vi "Assign switches.vi"(8 "error in (no error)":errorcluster, 10 "Channel Array In":T1=[{"Channel x"="x6", "Channel y"="y1"}, {"Channel x"="x2", "Channel y"="y5"}]) -> (0 "error out":errorcluster, 2 "Channel Array Out":T1=[{"Channel x"="xA6", "Channel y"="yA1"}, {"Channel x"="comB6", "Channel y"="chB6"}, {"Channel x"="comD1", "Channel y"="chD1"}, {"Channel x"="xA2", "Channel y"="yA5"}, {"Channel x"="comC2", "Channel y"="chC2"}, {"Channel x"="comD5", "Channel y"="chD5"}])   [LabVIEW 2016, in "pickering.lvclass"]
uses:
  pickering.lvclass
  Typedefs/Channels-Array.ctl
  Typedefs/Channel-Cluster.ctl
  Typedefs/ChannelX-ComboBox.ctl
  Typedefs/ChannelY-ComboBox.ctl
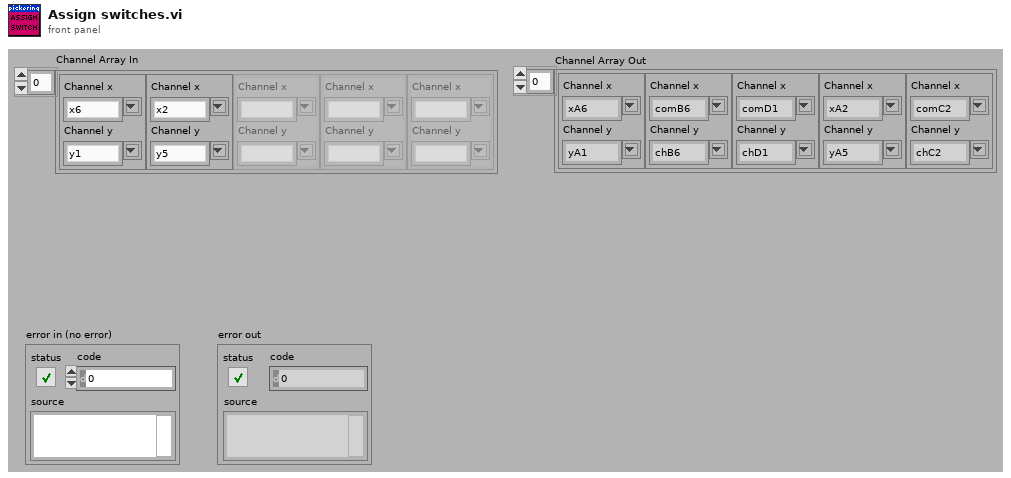
[diagram p1: front panel]
types:
  T1 = typedef "pickering.lvclass/Channels-Array.ctl" = T2[]
  T2 = typedef "pickering.lvclass/Channel-Cluster.ctl" = cluster{"Channel x":T3, "Channel y":T4}
  T3 = typedef "pickering.lvclass/ChannelX-ComboBox.ctl" = string
  T4 = typedef "pickering.lvclass/ChannelY-ComboBox.ctl" = string
  T5 = cluster{"result string":string, "result string":string}
  T6 = cluster{"result string":string, "result string":string}[]
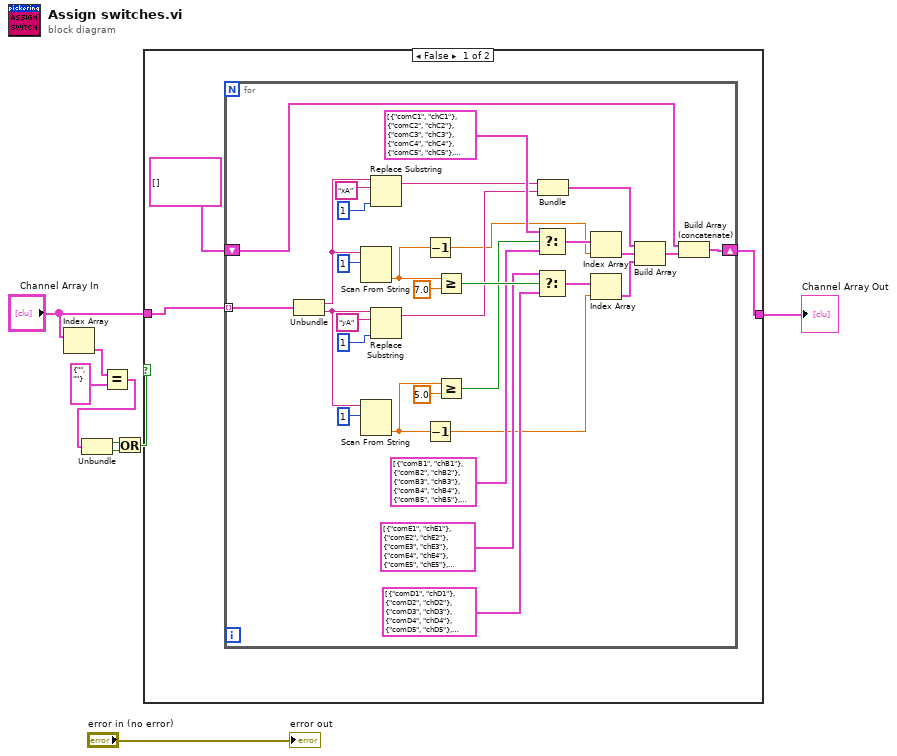
[diagram p0: block diagram]
diagram:
  n1 = Index Array(array="Channel Array In") -> (element=w7:T2)  [unwired: 1 in]
  n2 = Equal?(x=w7, y=cluster{"Channel x":string, "Channel y":string} {"Channel x"="", "Channel y"=""}) -> (x = y?=w5:cluster{"Channel x":bool, "Channel y":bool})
  n3 = Unbundle(w5) -> ("Channel x"=w4:bool, "Channel y"=w3:bool)
  n4 = Or(x=w4, y=w3) -> (x .or. y?=w2:bool)
  n5 = case shown="False" w2 {
    tunnel: "Channel Array In" -> [w11 w44]
    tunnel: [w12 w44] -> w9
    frame False {
      n6 = for {
        tunnel: w11 -> [w13] mode=indexing
        shift-right: [w15] -> w12
        shift-left: T1 [] -> [w14]
        n7 = Unbundle(w13) -> ("Channel x"=w18:T3, "Channel y"=w17:T4)
        n8 = Scan From String(input string=w18, initial scan location=u32 1) -> (output 1=w28:dbl)  [unwired: 3 in, 3 out]
        n9 = Scan From String(input string=w17, initial scan location=u32 1) -> (output 1=w26:dbl)  [unwired: 3 in, 3 out]
        n10 = Replace Substring(2:1 ("length (len. of substring)"), 4:"xA" ("substring (\"\")"), 5:w18) -> (1:w25:string)  [unwired: 1 in, 1 out]
        n11 = Replace Substring(2:1 ("length (len. of substring)"), 4:"yA" ("substring (\"\")"), 5:w17) -> (1:w24:string)  [unwired: 1 in, 1 out]
        n12 = Decrement(x=w28) -> (x-1=w21:dbl)
        n13 = Decrement(x=w26) -> (x-1=w22:dbl)
        n14 = Greater Or Equal?(x=w28, y=7.0) -> (x >= y?=w39:bool)
        n15 = Greater Or Equal?(x=w26, y=5.0) -> (x >= y?=w38:bool)
        n16 = Select(t=cluster{string, string}[] [{"comC1", "chC1"}, {"comC2", "chC2"}, {"comC3", "chC3"}, {"comC4", "chC4"}, {"comC5", "chC5"}, {"comC6", "chC6"}, {"comC7", "chC7"}, {"comC8", "chC8"}, {"comC9", "chC9"}, {"comC10", "chC10"}, {"comC11", "chC11"}, {"comC12", "chC12"}] ("Switch C"), s=w38, f=cluster{string, string}[] [{"comB1", "chB1"}, {"comB2", "chB2"}, {"comB3", "chB3"}, {"comB4", "chB4"}, {"comB5", "chB5"}, {"comB6", "chB6"}, {"comB7", "chB7"}, {"comB8", "chB8"}, {"comB9", "chB9"}, {"comB10", "chB10"}, {"comB11", "chB11"}, {"comB12", "chB12"}] ("Switch B")) -> (s? t:f=w27:cluster{string, string}[])
        n17 = Select(t=cluster{string, string}[] [{"comE1", "chE1"}, {"comE2", "chE2"}, {"comE3", "chE3"}, {"comE4", "chE4"}, {"comE5", "chE5"}, {"comE6", "chE6"}, {"comE7", "chE7"}, {"comE8", "chE8"}] ("Switch E"), s=w39, f=cluster{string, string}[] [{"comD1", "chD1"}, {"comD2", "chD2"}, {"comD3", "chD3"}, {"comD4", "chD4"}, {"comD5", "chD5"}, {"comD6", "chD6"}, {"comD7", "chD7"}, {"comD8", "chD8"}] ("Switch D")) -> (s? t:f=w29:cluster{string, string}[])
        n18 = Bundle("result string"=w25, "result string"=w24) -> (w23:T5)  [unwired: 1 in]
        n19 = Index Array(array=w27, index=w21) -> (element=w19:cluster{string, string})
        n20 = Index Array(array=w29, index=w22) -> (element=w20:cluster{string, string})
        n21 = Build Array(w23, w19, w20) -> (w16:T6)
        n22 = Build Array (concatenate)(w14, w16) -> (w15:T1)
      }
    }
    frame True {
    }
  }
  "Channel Array Out" <- w9
  "error out" <- "error in (no error)"
